vi "niRFUtil WFM Align Waveforms - Coarse (complex wfm).vi"(0 "Waveform In":T1 {"y" format="%.2f"; "dx" format="%^.2e"; "x0" format="%^.2e"}, 5 "Reference Waveform":T1 {"y" format="%.2f"; "dx" format="%^.2e"; "x0" format="%^.2e"}, 7 "Window Start, sec":dbl format="%^.2e", 9 "Window Duration, sec":dbl format="%^.2e") -> (4 "Waveform Out":T1 {"y" format="%.2f"; "dx" format="%^.2e"; "x0" format="%^.2e"})   [LabVIEW 2015, in "niRFUtil.lvlib"]
doc: "(c) Copyright 2006, National Instruments, Inc. This VI may not be duplicated, sold, or distributed without written consent from National Instruments."
uses:
  niRFUtil.lvlib
  Includes/niRFUtil INC Complex Waveform.ctl
  Includes/niRFUtil INC Complex Array.ctl
  niRFUtil WFM Complex Differential (complex wfm).vi
  niRFUtil WFM Parse Waveform - Duration (complex wfm).vi
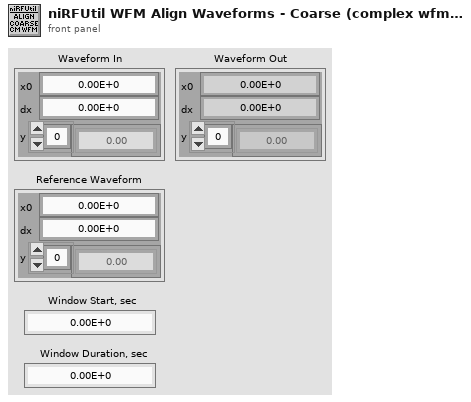
[diagram p1: front panel]
types:
  T1 = typedef "niRFUtil.lvlib/niRFUtil INC Complex Waveform.ctl" = cluster{"x0":dbl, "dx":dbl, "y":T2}
  T2 = typedef "niRFUtil.lvlib/niRFUtil INC Complex Array.ctl" = csg[]
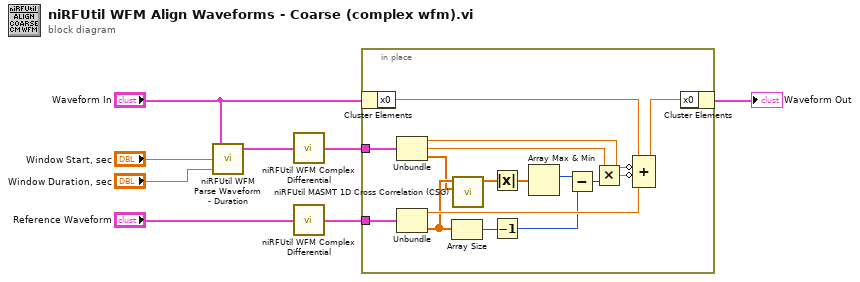
[diagram p0: block diagram]
diagram:
  n1 = call-poly "niRFUtil WFM Parse Waveform - Duration.vi"("Duration (Inf)"="Window Duration, sec", "Start (-Inf)"="Window Start, sec", "Waveform In"="Waveform In") -> ("Waveform Out"=w4:T1)  [unwired: 2 out]
  n2 = call-poly "niRFUtil WFM Complex Differential.vi"("Waveform In"=w4) -> ("Waveform Out"=w3:T1)  [unwired: 14 out]
  n3 = call-poly "niRFUtil WFM Complex Differential.vi"("Waveform In"="Reference Waveform") -> ("Waveform Out"=w1:T1)  [unwired: 14 out]
  n4 = in-place {
    in-place-border: w1 -> [w24]
    in-place-border: w3 -> [w23]
    n5 = in-place-cluster #1("Waveform In") -> ("x0"=w10:dbl)
    n6 = Unbundle(w23) -> ("x0"=w14:dbl, "dx"=w18:dbl, "y"=w11:T2)
    n7 = Unbundle(w24) -> ("x0"=w16:dbl, "y"=w12:T2)  [unwired: 1 out]
    n8 = Array Size(array=w12) -> (size(s)=w15:i32)
    n9 = call "niRFUtil MASMT 1D Cross Correlation (CSG).vi"("Y"=w11, "X"=w12) -> ("Rxy"=w22:csg[])  [unwired: 8 in, 1 out]
    n10 = Absolute Value(x=w22) -> (abs(x)=w21:sgl[])
    n11 = Decrement(x=w15) -> (x-1=w13:i32)
    n12 = Array Max & Min(array=w21) -> (max index (indices)=w20:i32)  [unwired: 3 out]
    n13 = Subtract(x=w20, y=w13) -> (x-y=w19:i32)
    n14 = Multiply(x=w18, y=w19) -> (x*y=w17:dbl)
    n15 = Compound Arithmetic op=ADD(w10, invert w14, invert w17, w16) -> (w9:dbl)
    n16 = in-place-cluster #1("x0"=w9) -> (→"Waveform Out":T1)
  }
